vi "cRIO_EPTx_FPGA.vi"() -> ()   [LabVIEW 2020]
uses:
  <vilib>/Platform/TimedLoop/XDataNode/wakeup.ctl
  <vilib>/Platform/TimedLoop/XDataNode/XDNodeRunTimeDep.lvlib
  <vilib>/Platform/TimedLoop/XDataNode/nitl_modes.ctl
  <vilib>/Platform/TimedLoop/XDataNode/timing_clust.ctl
  <vilib>/Platform/TimedLoop/XDataNode/XDataNode.xnode
  <vilib>/eio/EIONode/EIONode.xnode
  <vilib>/Powertrain Controls/Device Drivers/Engine Position Tracking/EPTx/RevA/FPGA/Controls/EPTxAAPControl.ctl
  <vilib>/Powertrain Controls/Device Drivers/Engine Position Tracking/EPTx/RevA/FPGA/EPTx - RevA - FPGA.lvlib
  <vilib>/Powertrain Controls/Device Drivers/Engine Position Tracking/EPTx/RevA/FPGA/Controls/Patterns.ctl
  <vilib>/Powertrain Controls/Device Drivers/Engine Position Tracking/EPTx/RevA/FPGA/Controls/EPTxPatternConfig.ctl
  <vilib>/Powertrain Controls/Device Drivers/Engine Position Tracking/EPTx/RevA/FPGA/Controls/EPTxControl.ctl
  <vilib>/rvi/eio/common/nirviEmuTemplateMethod_errors.vi
  <vilib>/Powertrain Controls/Device Drivers/Engine Position Tracking/EPTx/RevA/FPGA/Controls/EPTxSignals.ctl
  <vilib>/Powertrain Controls/Device Drivers/Engine Position Tracking/EPTx/RevA/FPGA/Controls/EPTxSimulatorConfig.ctl
  <vilib>/Powertrain Controls/Device Drivers/Engine Position Tracking/EPTx/RevA/FPGA/Controls/EPTxDebug.ctl
  <vilib>/Powertrain Controls/Device Drivers/Engine Position Tracking/EPTx/RevA/FPGA/Controls/EPTxTooth.ctl
  <vilib>/Powertrain Controls/Device Drivers/Engine Position Tracking/EPTx/RevA/FPGA/Controls/EPTxSupervisor.ctl
  <vilib>/Powertrain Controls/Device Drivers/Engine Position Tracking/EPTx/RevA/FPGA/Controls/EPTxConfig.ctl
panel:
  out "OpenWinSig":bool
  in  "Delay[tick]":u32
  out "Injection_Sig":bool
  out "CAN_Trigger":bool
  out "Speed_Output":fxp<+/-,32,16>
  out "Cylinder_Number":u8
  in  "OpWin_Enable6":bool
  in  "OpWin_RisingCAD6":fxp<+/-,32,16>=540.0
  in  "OpWin_FallingCAD6":fxp<+/-,32,16>=600.0
  in  "Cylinder6_H_R [CAD]":fxp<+/-,32,16>
  in  "Cylinder6_H_F [CAD]":fxp<+/-,32,16>
  in  "OpWin_Enable5":bool
  in  "OpWin_RisingCAD5":fxp<+/-,32,16>=300.0
  in  "OpWin_FallingCAD5":fxp<+/-,32,16>=360.0
  in  "Cylinder5_H_R [CAD]":fxp<+/-,32,16>
  in  "Cylinder5_H_F [CAD]":fxp<+/-,32,16>
  in  "OpWin_Enable4":bool
  in  "OpWin_RisingCAD4":fxp<+/-,32,16>=60.0
  in  "OpWin_FallingCAD4":fxp<+/-,32,16>=120.0
  in  "Cylinder4_H_R [CAD]":fxp<+/-,32,16>
  in  "Cylinder4_H_F [CAD]":fxp<+/-,32,16>
  in  "OpWin_Enable3":bool
  in  "OpWin_RisingCAD3":fxp<+/-,32,16>=420.0
  in  "OpWin_FallingCAD3":fxp<+/-,32,16>=480.0
  in  "Cylinder3_H_R [CAD]":fxp<+/-,32,16>
  in  "Cylinder3_H_F [CAD]":fxp<+/-,32,16>
  in  "OpWin_Enable2":bool
  in  "OpWin_RisingCAD2":fxp<+/-,32,16>=660.0
  in  "OpWin_FallingCAD2":fxp<+/-,32,16>=720.0
  in  "Cylinder2_H_R [CAD]":fxp<+/-,32,16>
  in  "Cylinder2_H_F [CAD]":fxp<+/-,32,16>
  out "Watchdog Error":bool
  in  "Cylinder1_H_F [CAD]":fxp<+/-,32,16>
  in  "Cylinder1_H_R [CAD]":fxp<+/-,32,16>
  in  "Aux 4":fxp<+/-,32,16>
  in  "Aux 3":fxp<+/-,32,16>
  in  "Aux 2":fxp<+/-,32,16>
  in  "Aux 1":fxp<+/-,32,16>
  in  "OpWin_FallingCAD1":fxp<+/-,32,16>=240.0
  in  "OpWin_RisingCAD1":fxp<+/-,32,16>=180.0
  in  "Sim Rate":fxp<+/-,16,7>
  in  "Watchdog":bool
  in  "Sim Enable":bool
  in  "Clear Errors":bool
  in  "Sync Enable":bool
  in  "OpWin_Enable1":bool
  in  "Aux 4 State":bool
  in  "Aux 3 State":bool
  in  "Aux 2 State":bool
  in  "Aux 1 State":bool
  in  "Primary State":bool
  in  "Primary":fxp<+/-,32,16>
  in  "Address":fxp<+/-,32,16>
  out "AvgSpeed":fxp<+/-,32,16>
  out "CADRate":fxp<+/-,32,16>
  out "HistoryCAD":fxp<+/-,32,16>
  out "MaxCAD":fxp<+/-,32,16>
  out "CurrentCAD":fxp<+/-,32,16>
  out "EndCAD":fxp<+/-,32,16>
  out "StartCAD":fxp<+/-,32,16>
  out "CycleCount":fxp<+/-,64,32>
  out "Forward":bool
  out "Tooth":bool
  out "Sync 2":bool
  out "Aux Warning":bool
  out "Pattern Error":bool
  out "Ratio Error":bool
  out "Overflow":bool
  out "Stall":bool
  out "Rcvg Primary":bool
  out "Config":bool
  out "Sync":bool
  in  "EPTxConfig":T1
  out "EPTxSupervisor_FPGA":T2
  out "EPTxSignals":T3
  out "EPTxTooth":T4
  out "EPTxDebug":T5
  in  "EPTxSimulatorConfig":T6
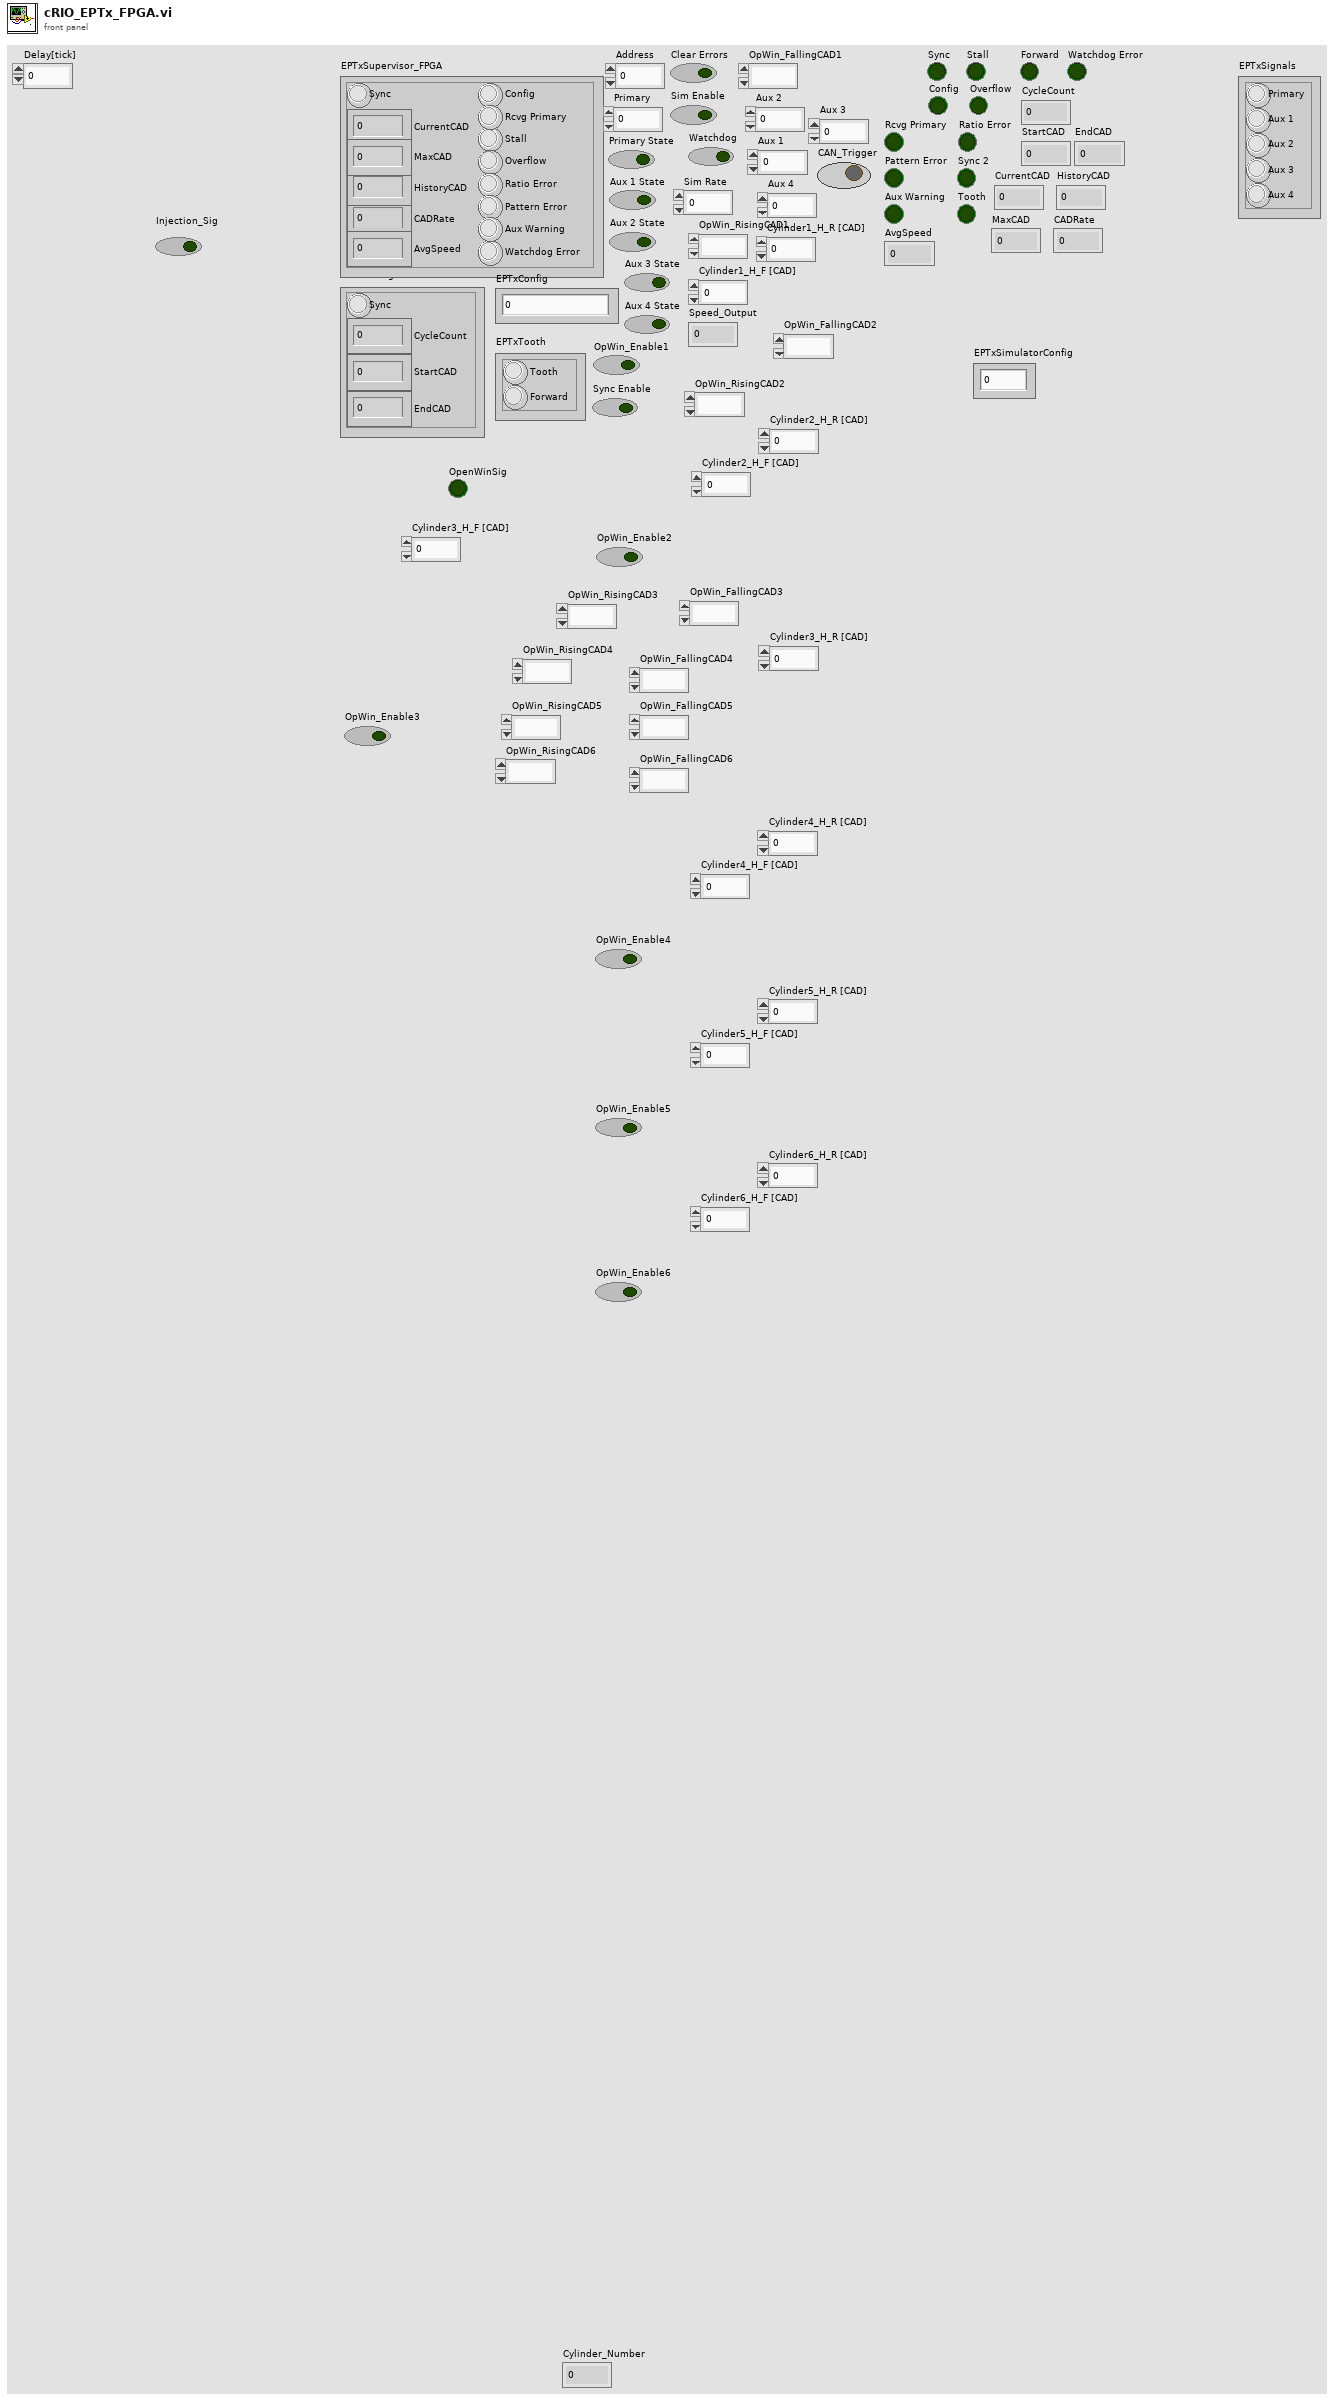
[diagram p1: front panel]
types:
  T1 = typedef "EPTx - RevA - FPGA.lvlib/EPTxConfig.ctl" = u64
  T2 = typedef "EPTx - RevA - FPGA.lvlib/EPTxSupervisor.ctl" = cluster{"Sync":bool, "CurrentCAD":fxp<+,18,11>, "MaxCAD":fxp<+,11,11>, "HistoryCAD":fxp<+,11,11>, "CADRate":fxp<+,22,8>, "AvgSpeed":fxp<+,17,15>, "Config":bool, "Rcvg Primary":bool, "Stall":bool, "Overflow":bool, "Ratio Error":bool, "Pattern Error":bool, "Aux Warning":bool, "Watchdog Error":bool}
  T3 = typedef "EPTx - RevA - FPGA.lvlib/EPTxSignals.ctl" = cluster{"Primary":bool, "Aux 1":bool, "Aux 2":bool, "Aux 3":bool, "Aux 4":bool}
  T4 = typedef "EPTx - RevA - FPGA.lvlib/EPTxTooth.ctl" = cluster{"Tooth":bool, "Forward":bool}
  T5 = typedef "EPTx - RevA - FPGA.lvlib/EPTxDebug.ctl" = cluster{"Sync":bool, "CycleCount":fxp<+,8,8>, "StartCAD":fxp<+,18,11>, "EndCAD":fxp<+,18,11>}
  T6 = typedef "EPTx - RevA - FPGA.lvlib/EPTxSimulatorConfig.ctl" = u32
  T7 = typedef "EPTx - RevA - FPGA.lvlib/EPTxAAPControl.ctl" = cluster{"Enable":bool, "RisingCAD":fxp<+,18,11>, "FallingCAD":fxp<+,18,11>}
  T8 = typedef "XDNodeRunTimeDep.lvlib/timing_clust.ctl" = cluster{"Expected End [f-1]":u64, "Actual End [f-1]":u64, "Finished Late? [f-1]":bool, "Expected End [i-1]":u64, "Actual End [i-1]":u64, "Finished Late? [i-1]":bool, "Expected Start [i]":u64, "Actual Start [i]":u64, "Expected Start [f]":u64, "Actual Start [f]":u64, "Source Name":string, "Structure Name":string, "Period":i64, "Deadline":i64, "Offset":i64, "Start":i64, "Priority":i32, "Timeout":i32, "Mode":T9, "Wakeup Reason":T10, "Error":errorcluster, "Source Type":string, "Secondary Source Type":string, "Global End Time":u64, "Global Start Time":u64, "Frame Duration":u64, "Iteration Duration":u64, "Assigned CPU":i32, "I/O Scan Engine Mode":u32}
  T9 = typedef "XDNodeRunTimeDep.lvlib/nitl_modes.ctl" = enum32{"No Change", "Process missed periods, maintain original phase", "Discard missed periods, maintain original phase", "Process missed periods, ignore original phase", "Discard missed periods, ignore original phase"}
  T10 = typedef "XDNodeRunTimeDep.lvlib/wakeup.ctl" = enum32{"Normal", "Aborted", "Asynchronous wakeup", "Timing source error", "Timed loop error", "Timeout"}
  T11 = typedef "EPTx - RevA - FPGA.lvlib/EPTxControl.ctl" = cluster{"Sync Enable":bool, "Clear Errors":bool, "Sim Enable":bool, "Sim Rate":fxp<+,24,6>, "Watchdog":bool}
  T12 = typedef "EPTx - RevA - FPGA.lvlib/Patterns.ctl" = cluster{"Primary":fxp<+,19,12>, "Primary State":bool, "Aux 1":fxp<+,19,12>, "Aux 1 State":bool, "Aux 2":fxp<+,19,12>, "Aux 2 State":bool, "Aux 3":fxp<+,19,12>, "Aux 3 State":bool, "Aux 4":fxp<+,19,12>, "Aux 4 State":bool}
  T13 = typedef "EPTx - RevA - FPGA.lvlib/EPTxPatternConfig.ctl" = cluster{"Address":fxp<+,14,14>, "Pattern":T12}
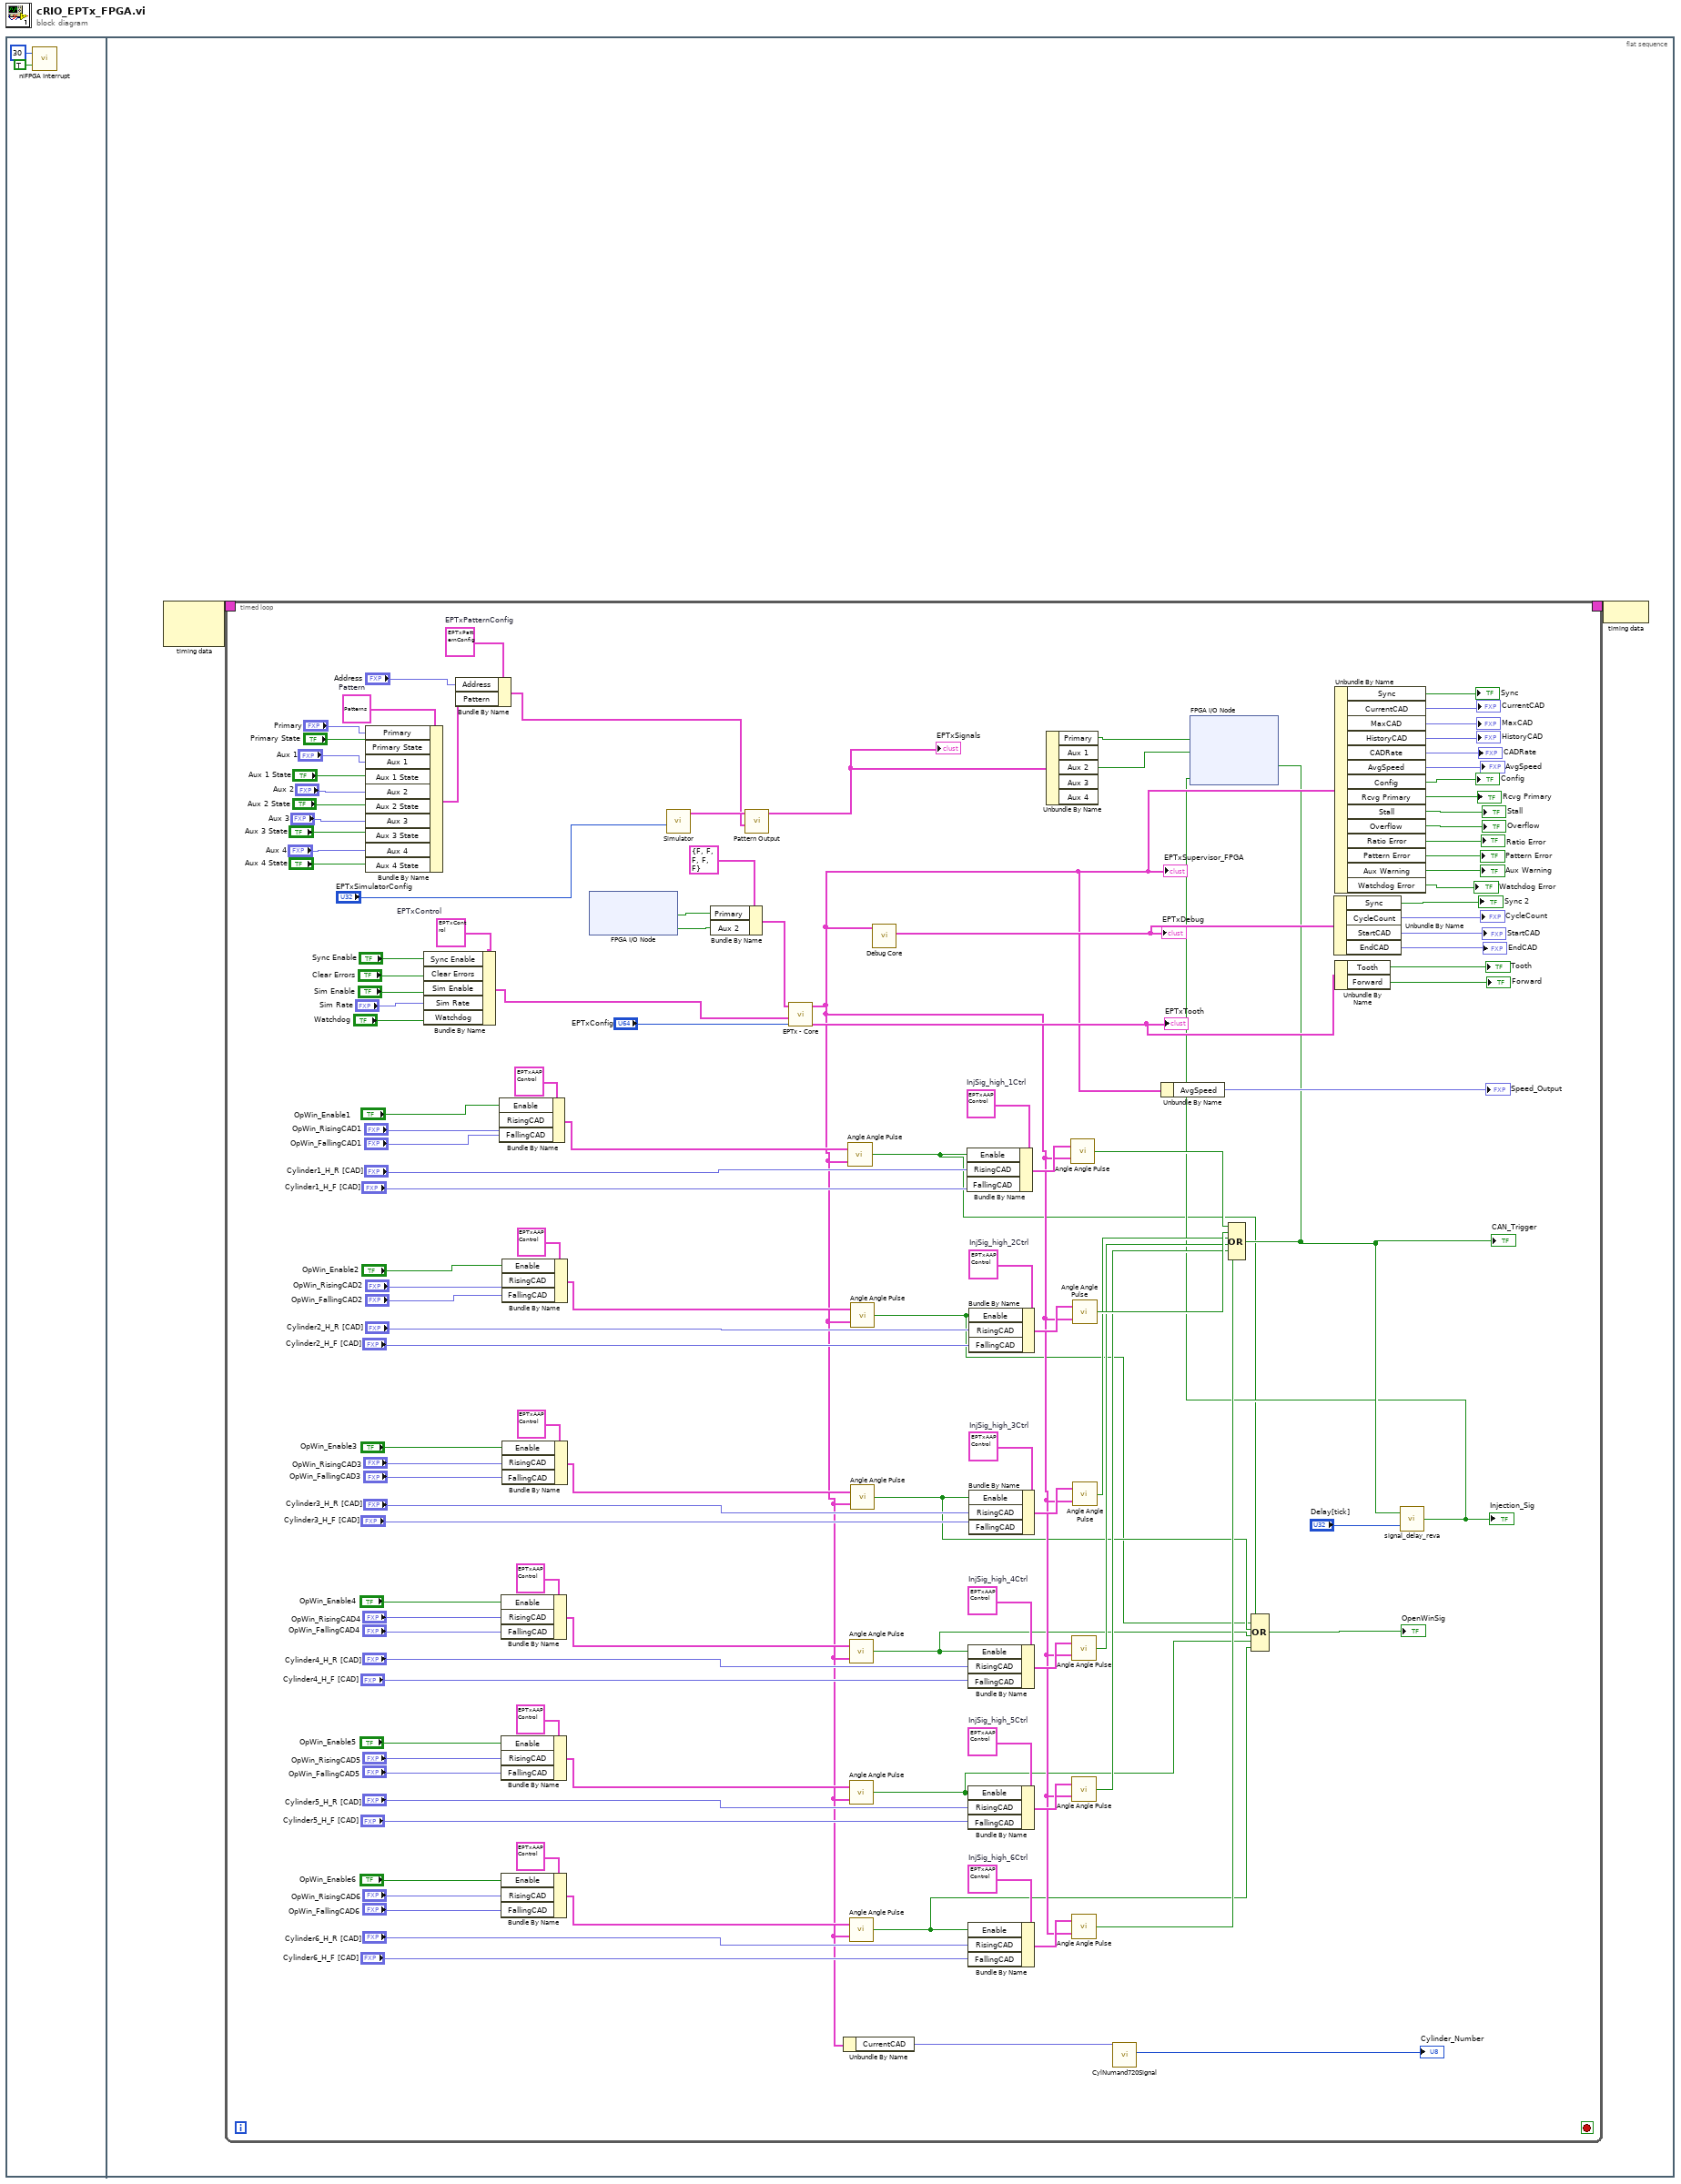
[diagram p0: block diagram]
diagram:
  n1 = flat-sequence {
    frame #0 {
      n2 = call <vilib>:"niFPGA Interrupt.vi"("Wait Until Cleared (F)"=TRUE, "IRQ Number (0)"=u8 30) -> ()  [unwired: 1 in]
    }
    frame #1 {
      n3 = node-c288() -> (w4:T8)  [unwired: 2 in]
      n4 = timed-loop {
        timing: w4 -> [_]
        timing-out: [_] -> w3
        stop <- _ stop-if-true
        w28 = T7 {"Enable"=FALSE, "RisingCAD"=0.0, "FallingCAD"=0.0}  # InjSig_high_6Ctrl
        w43 = T7 {"Enable"=FALSE, "RisingCAD"=0.0, "FallingCAD"=0.0}  # InjSig_high_5Ctrl
        w46 = T7 {"Enable"=FALSE, "RisingCAD"=0.0, "FallingCAD"=0.0}  # InjSig_high_4Ctrl
        w63 = T7 {"Enable"=FALSE, "RisingCAD"=0.0, "FallingCAD"=0.0}  # InjSig_high_3Ctrl
        w67 = T7 {"Enable"=FALSE, "RisingCAD"=0.0, "FallingCAD"=0.0}  # InjSig_high_2Ctrl
        w117 = T11 {"Sync Enable"=FALSE, "Clear Errors"=FALSE, "Sim Enable"=FALSE, "Sim Rate"=0.0, "Watchdog"=FALSE}  # EPTxControl
        w122 = T12 {"Primary"=0.0, "Primary State"=FALSE, "Aux 1"=0.0, "Aux 1 State"=FALSE, "Aux 2"=0.0, "Aux 2 State"=FALSE, "Aux 3"=0.0, "Aux 3 State"=FALSE, "Aux 4"=0.0, "Aux 4 State"=FALSE}  # Pattern
        w123 = T13 {"Address"=0.0, "Pattern"={"Primary"=0.0, "Primary State"=FALSE, "Aux 1"=0.0, "Aux 1 State"=FALSE, "Aux 2"=0.0, "Aux 2 State"=FALSE, "Aux 3"=0.0, "Aux 3 State"=FALSE, "Aux 4"=0.0, "Aux 4 State"=FALSE}}  # EPTxPatternConfig
        w126 = T7 {"Enable"=FALSE, "RisingCAD"=0.0, "FallingCAD"=0.0}  # InjSig_high_1Ctrl
        n5 = Bundle By Name(cluster=w122, "Primary"="Primary", "Primary State"="Primary State", "Aux 1"="Aux 1", "Aux 1 State"="Aux 1 State", "Aux 2"="Aux 2", "Aux 2 State"="Aux 2 State", "Aux 3"="Aux 3", "Aux 3 State"="Aux 3 State", "Aux 4"="Aux 4", "Aux 4 State"="Aux 4 State") -> (w121:T12)
        n6 = Bundle By Name(cluster=w117, "Sync Enable"="Sync Enable", "Clear Errors"="Clear Errors", "Sim Enable"="Sim Enable", "Sim Rate"="Sim Rate", "Watchdog"="Watchdog") -> (w116:T11)
        n7 = Bundle By Name(cluster=w123, "Address"="Address", "Pattern"=w121) -> (w120:T13)
        n8 = Bundle By Name(cluster=T7 {"Enable"=FALSE, "RisingCAD"=0.0, "FallingCAD"=0.0} ("AAPControl_1str"), "Enable"="OpWin_Enable1", "RisingCAD"="OpWin_RisingCAD1", "FallingCAD"="OpWin_FallingCAD1") -> (w118:T7)
        n9 = Bundle By Name(cluster=T7 {"Enable"=FALSE, "RisingCAD"=0.0, "FallingCAD"=0.0} ("AAPControl_1str"), "Enable"="OpWin_Enable4", "RisingCAD"="OpWin_RisingCAD4", "FallingCAD"="OpWin_FallingCAD4") -> (w48:T7)
        n10 = Bundle By Name(cluster=T7 {"Enable"=FALSE, "RisingCAD"=0.0, "FallingCAD"=0.0} ("AAPControl_1str"), "Enable"="OpWin_Enable5", "RisingCAD"="OpWin_RisingCAD5", "FallingCAD"="OpWin_FallingCAD5") -> (w41:T7)
        n11 = Bundle By Name(cluster=T7 {"Enable"=FALSE, "RisingCAD"=0.0, "FallingCAD"=0.0} ("AAPControl_1str"), "Enable"="OpWin_Enable6", "RisingCAD"="OpWin_RisingCAD6", "FallingCAD"="OpWin_FallingCAD6") -> (w30:T7)
        n12 = Bundle By Name(cluster=T7 {"Enable"=FALSE, "RisingCAD"=0.0, "FallingCAD"=0.0} ("AAPControl_1str"), "Enable"="OpWin_Enable2", "RisingCAD"="OpWin_RisingCAD2", "FallingCAD"="OpWin_FallingCAD2") -> (w69:T7)
        n13 = Bundle By Name(cluster=T7 {"Enable"=FALSE, "RisingCAD"=0.0, "FallingCAD"=0.0} ("AAPControl_1str"), "Enable"="OpWin_Enable3", "RisingCAD"="OpWin_RisingCAD3", "FallingCAD"="OpWin_FallingCAD3") -> (w61:T7)
        n14 = xnode "FPGA I/O Node"() -> ("Mod7/DIO0"=w16:bool, "Mod7/DIO1"=w15:bool)  [unwired: 2 in, 2 out]
        n15 = call <vilib>:"Simulator.vi"("EPTxSimulatorConfig"="EPTxSimulatorConfig") -> ("EPTxSupervisor"=w131:T2)  [unwired: 10 in]
        n16 = Bundle By Name(cluster=T3 {"Primary"=FALSE, "Aux 1"=FALSE, "Aux 2"=FALSE, "Aux 3"=FALSE, "Aux 4"=FALSE} ("EPTxSignals"), "Primary"=w16, "Aux 2"=w15) -> (w17:T3)
        n17 = call <vilib>:"Pattern Output.vi"("EPTxPatternConfig"=w120, "EPTxSupervisor"=w131) -> ("PatternOutput"=w129:T3)  [unwired: 9 in]
        "EPTxSignals" <- w129
        n18 = call <vilib>:"EPTx - Core.vi"("EPTxConfig"="EPTxConfig", "EPTxControl"=w116, "EPTxSignals"=w17) -> ("EPTxTooth"=w124:T4, "EPTxSupervisor"=w21:T2)  [unwired: 7 in]
        "EPTxSupervisor_FPGA" <- w21
        "EPTxTooth" <- w124
        n19 = Unbundle By Name(w21) -> ("CurrentCAD"=w22:fxp<+,18,11>)
        n20 = call <vilib>:"Angle Angle Pulse.vi"("EPTxSupervisor"=w21, "AAPControl"=w118) -> ("AAP"=w6:bool)
        n21 = call <vilib>:"Angle Angle Pulse.vi"("EPTxSupervisor"=w21, "AAPControl"=w48) -> ("AAP"=w9:bool)
        n22 = call <vilib>:"Angle Angle Pulse.vi"("EPTxSupervisor"=w21, "AAPControl"=w41) -> ("AAP"=w10:bool)
        n23 = call <vilib>:"Angle Angle Pulse.vi"("EPTxSupervisor"=w21, "AAPControl"=w30) -> ("AAP"=w11:bool)
        n24 = call <vilib>:"Angle Angle Pulse.vi"("EPTxSupervisor"=w21, "AAPControl"=w69) -> ("AAP"=w7:bool)
        n25 = call <vilib>:"Angle Angle Pulse.vi"("EPTxSupervisor"=w21, "AAPControl"=w61) -> ("AAP"=w8:bool)
        n26 = call <vilib>:"Debug Core.vi"("EPTxSupervisor"=w21) -> ("EPTxDebug"=w125:T5)  [unwired: 10 in]
        "EPTxDebug" <- w125
        n27 = Bundle By Name(cluster=w126, "Enable"=w6, "RisingCAD"="Cylinder1_H_R [CAD]", "FallingCAD"="Cylinder1_H_F [CAD]") -> (w127:T7)
        n28 = Bundle By Name(cluster=w46, "Enable"=w9, "RisingCAD"="Cylinder4_H_R [CAD]", "FallingCAD"="Cylinder4_H_F [CAD]") -> (w45:T7)
        n29 = Bundle By Name(cluster=w43, "Enable"=w10, "RisingCAD"="Cylinder5_H_R [CAD]", "FallingCAD"="Cylinder5_H_F [CAD]") -> (w44:T7)
        n30 = Bundle By Name(cluster=w28, "Enable"=w11, "RisingCAD"="Cylinder6_H_R [CAD]", "FallingCAD"="Cylinder6_H_F [CAD]") -> (w27:T7)
        n31 = Bundle By Name(cluster=w67, "Enable"=w7, "RisingCAD"="Cylinder2_H_R [CAD]", "FallingCAD"="Cylinder2_H_F [CAD]") -> (w66:T7)
        n32 = Bundle By Name(cluster=w63, "Enable"=w8, "RisingCAD"="Cylinder3_H_R [CAD]", "FallingCAD"="Cylinder3_H_F [CAD]") -> (w64:T7)
        n33 = Unbundle By Name(w129) -> ("Primary"=w128:bool, "Aux 2"=w19:bool)  [unwired: 3 out]
        n34 = call <vilib>:"Angle Angle Pulse.vi"("EPTxSupervisor"=w21, "AAPControl"=w127) -> ("AAP"=w65:bool)
        n35 = call <vilib>:"Angle Angle Pulse.vi"("EPTxSupervisor"=w21, "AAPControl"=w45) -> ("AAP"=w26:bool)
        n36 = call <vilib>:"Angle Angle Pulse.vi"("EPTxSupervisor"=w21, "AAPControl"=w44) -> ("AAP"=w25:bool)
        n37 = call <vilib>:"Angle Angle Pulse.vi"("EPTxSupervisor"=w21, "AAPControl"=w27) -> ("AAP"=w24:bool)
        n38 = call <vilib>:"Angle Angle Pulse.vi"("EPTxSupervisor"=w21, "AAPControl"=w66) -> ("AAP"=w55:bool)
        n39 = call <vilib>:"Angle Angle Pulse.vi"("EPTxSupervisor"=w21, "AAPControl"=w64) -> ("AAP"=w54:bool)
        n40 = call "CylNumand720Signal.vi"("CurrentCAD"=w22) -> ("数值输入控件"=→"Cylinder_Number":u8)  [unwired: 10 in]
        n41 = Unbundle By Name(w21) -> ("AvgSpeed"=→"Speed_Output":fxp<+,17,15>)
        n42 = Compound Arithmetic op=OR ("复合运算")(w65, w55, w54, w26, w25, w24) -> (w14:bool)
        "CAN_Trigger" <- w14
        n43 = Compound Arithmetic op=OR ("复合运算")(w6, w7, w8, w9, w10, w11) -> (→"OpenWinSig":bool)
        n44 = Unbundle By Name(w125) -> ("Sync"=→"Sync 2":bool, "CycleCount"=→"CycleCount":fxp<+,8,8>, "StartCAD"=→"StartCAD":fxp<+,18,11>, "EndCAD"=→"EndCAD":fxp<+,18,11>)
        n45 = Unbundle By Name(w21) -> ("Sync"=→"Sync":bool, "CurrentCAD"=→"CurrentCAD":fxp<+,18,11>, "MaxCAD"=→"MaxCAD":fxp<+,11,11>, "HistoryCAD"=→"HistoryCAD":fxp<+,11,11>, "CADRate"=→"CADRate":fxp<+,22,8>, "AvgSpeed"=→"AvgSpeed":fxp<+,17,15>, "Config"=→"Config":bool, "Rcvg Primary"=→"Rcvg Primary":bool, "Stall"=→"Stall":bool, "Overflow"=→"Overflow":bool, "Ratio Error"=→"Ratio Error":bool, "Pattern Error"=→"Pattern Error":bool, "Aux Warning"=→"Aux Warning":bool, "Watchdog Error"=→"Watchdog Error":bool)
        n46 = Unbundle By Name(w124) -> ("Tooth"=→"Tooth":bool, "Forward"=→"Forward":bool)
        n47 = call <vilib>:"signal_delay_reva.vi"("Delay"="Delay[tick]", "InpSig"=w14) -> ("OutSig"=w12:bool)
        "Injection_Sig" <- w12
        n48 = xnode "FPGA I/O Node"("Mod6/DIO0"=w128, "Mod6/DIO1"=w19, "Mod6/DIO2"=w14, "Mod6/DIO3"=w12) -> ()  [unwired: 4 in, 4 out]
      }
      n49 = node-c288(w3) -> ()
    }
  }
